vi "Spartan Server.vi"() -> ()   [LabVIEW 2011]
uses:
  server lib/Spartan Version.vi
  http/Spartan HTTP Server Globals.vi
  Addons/internet/http/http0.llb/HTTP LVHTTP Global.vi
  OpenG.LIB/file/file.llb/Convert File Extension (Path)__ogtk.vi
  server lib/Spartan CONFIG Global.vi
panel:
  out "Uptime":dbl
  in  "clear":bool
  in  "?":bool
  out "DD Queue":i32
  out "ver":string
  in  "Show Log":bool
  out "tall":bool
  out "wide":bool
  out "narrow":bool
  out "Log":string
  out "short":bool
  out "time up":string
  out "time":string
  in  "do stop":bool
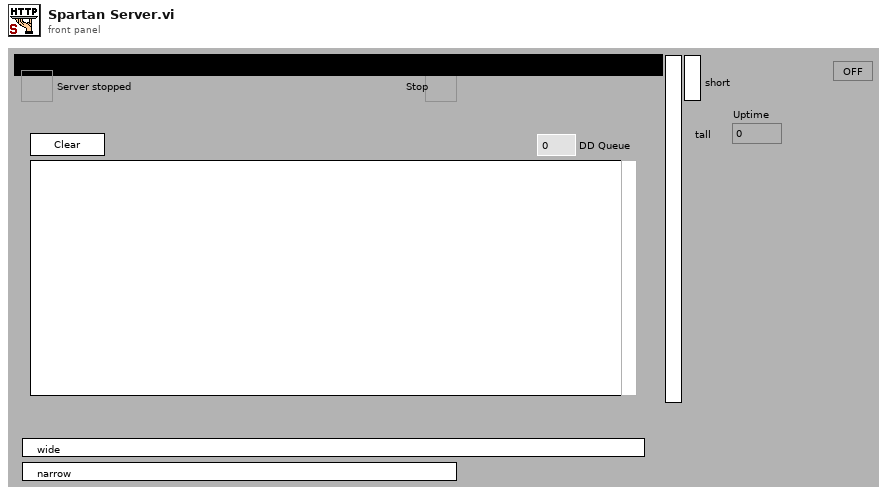
[diagram p1: front panel]
types:
  T1 = enum32{"Invalid", "Standard", "Closed", "Hidden", "Minimized", "Maximized"}
  T2 = enum32{"SW_SHOWDEFAULT", "SW_FORCEMINIMIZE", "SW_HIDE", "SW_MAXIMIZE", "SW_RESTORE", "SW_SHOW", "SW_SHOWMAXIMIZED", "SW_SHOWMINIMIZED", "SW_SHOWMINNOACTIVE", "SW_SHOWNA", "SW_SHOWNOACTIVATE", "SW_SHOWNORMAL"}
  T3 = typedef "OGAB Version.ctl" = cluster{"Version":string, "Build Number":u32, "Build Date/Time":dbl}
  T4 = typedef "DIAdem Queues.ctl" = cluster{"DIAdem Queue":refnum<queue>, "Datasheet Queue":refnum<queue>, "Runtest Queue":refnum<queue>}
  T5 = typedef "DIAdem Reference.ctl" = cluster{"ToCommand Reference":refnum<k7>, "ToDataSheet Reference":refnum<k7>}
  T6 = typedef "Semaphore RefNum" = refnum<k1>
  T7 = typedef "hWnd.ctl" = refnum<k1>
  T8 = typedef "siwutil32.ctl" = refnum<k7>
  T9 = typedef "LVRectTypeDef.ctl" = cluster{"left":i16, "top":i16, "right":i16, "bottom":i16}
  T10 = typedef "sizeaction.ctl" = enum32{"Minimized", "Maximized", "Resized"}
  T11 = typedef "Rendezvous RefNum" = refnum<k1>
  T12 = typedef "Keyed Array.ctl" = cluster{"keys":string[], "values":string[]}
  T13 = enum32{"invalid app kind", "Development System", "Run Time System", "Student Edition", "Embedded LabVIEW", "Evaluation", "Custom"}
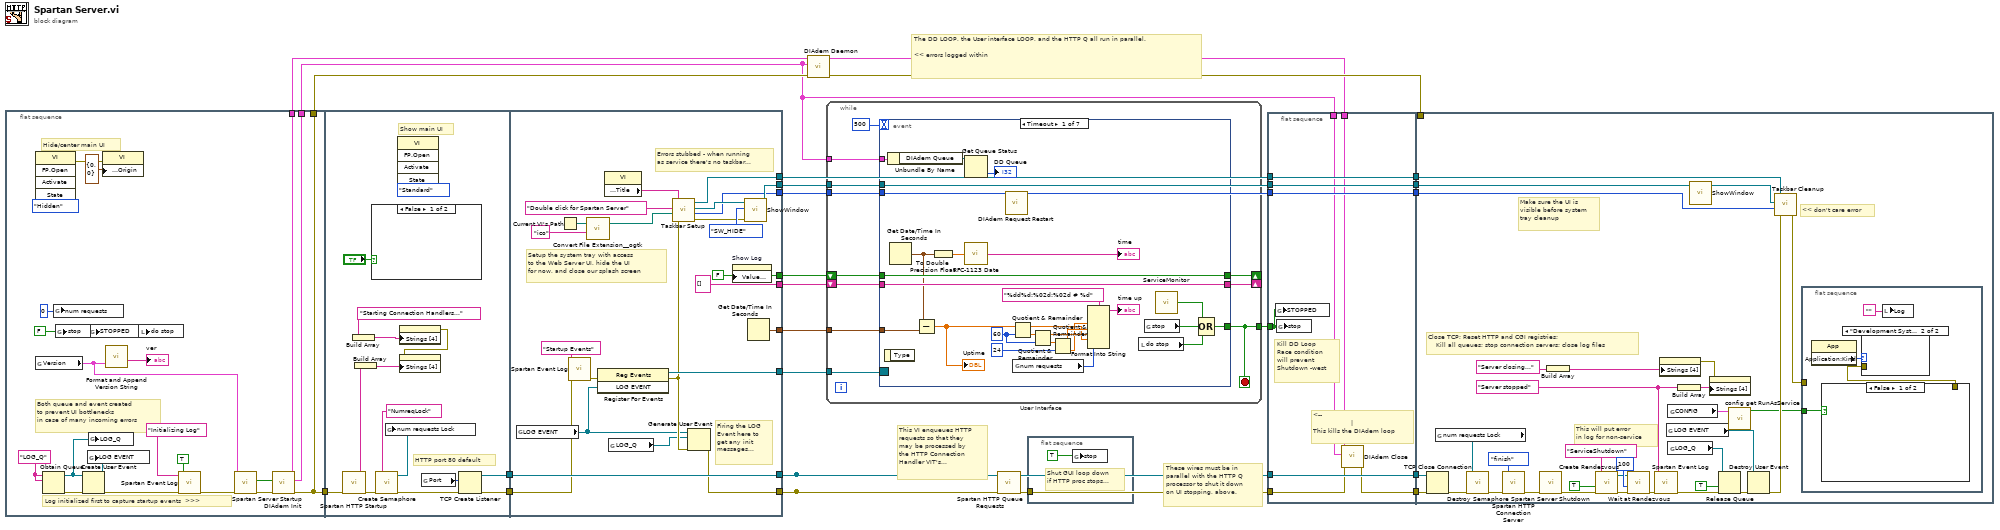
[diagram p0: block diagram]
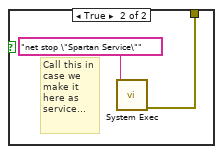
[diagram p2: hidden frame]
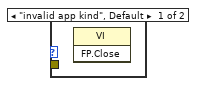
[diagram p3: hidden frame]
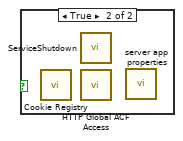
[diagram p4: hidden frame]
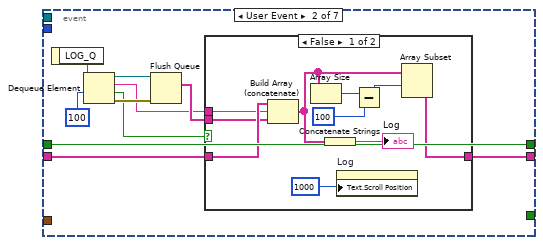
[diagram p5: hidden frame]
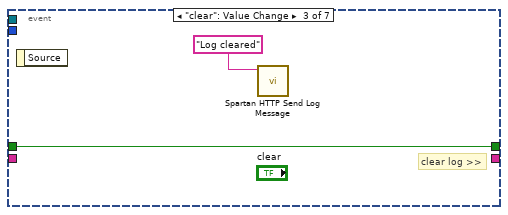
[diagram p7: hidden frame]
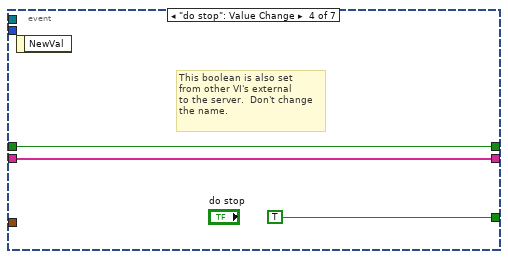
[diagram p8: hidden frame]
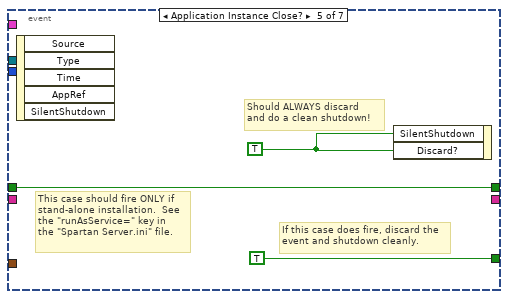
[diagram p9: hidden frame]
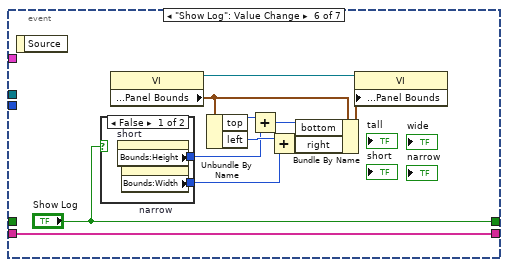
[diagram p10: hidden frame]
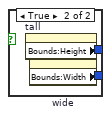
[diagram p11: hidden frame]
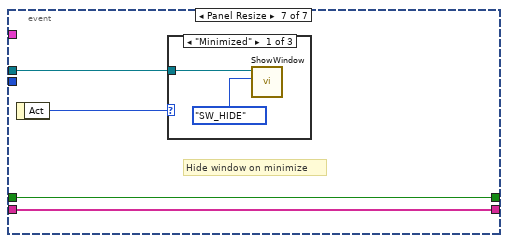
[diagram p12: hidden frame]
diagram:
  # "The DD LOOP, the User interface LOOP, and the HTTP Q all run in parallel.  \n\n<< errors logged within"
  # "These wires must be in\nparallel with the HTTP Q\nprocessor to shut it down\non UI stopping, above."
  # "This VI enqueues HTTP\nrequests so that they\nmay be processed by\nthe HTTP Connection\nHandler VIT's..."
  n1 = flat-sequence {
    tunnel: [w40] -> w12
    tunnel: [w42] -> w1
    tunnel: [w41] -> w3
    tunnel: [w40] -> w11
    tunnel: w12 -> [w50]
    tunnel: [w53] -> w18
    tunnel: [w51] -> w17
    tunnel: [w73] -> w22
    tunnel: [w81] -> w16
    tunnel: [w62] -> w13
    tunnel: [w80] -> w23
    tunnel: [w68] -> w10
    tunnel: w18 -> [w81]
    tunnel: [w76] -> w20
    tunnel: [w75] -> w21
    tunnel: [w74] -> w19
    tunnel: w17 -> [w61]
    tunnel: [string[] []] -> w14
    frame #0 {
      w32 = FALSE
      w36 = "LOG_Q"
      # "Hide/center main UI"
      # "Log initialized first to capture startup events  >>>"
      # "Both queue and event created\nto prevent UI bottlenecks\nin case of many incoming errors"
      n2 = invoke class="VI" method="FP.Open"("State"=T1."Hidden") -> (error out=w37:errorcluster)  [unwired: 4 in, 4 out]
      n3 = global read "Spartan Version.vi" "Version"() -> (w26:T3)
      n4 = Obtain Queue(name (unnamed)=w36, element data type=w36) -> (queue out=w33:refnum<queue>, error out=w35:errorcluster)  [unwired: 3 in, 1 out]
      n5 = global write "Spartan HTTP Server Globals.vi" "num requests"(u32 0 ("num requests")) -> ()
      n6 = global write "Spartan HTTP Server Globals.vi" "stop"(w32) -> ()
      n7 = Create User Event(user event datatype=w33, error in=w35) -> (user event=w34:refnum<user-event>, error out=w27:errorcluster)
      n8 = global write "Spartan HTTP Server Globals.vi" "LOG EVENT"(w34) -> ()
      n9 = global write "Spartan HTTP Server Globals.vi" "LOG_Q"(w33) -> ()
      n10 = global write "Spartan Version.vi" "STOPPED"(w32) -> ()
      n11 = property class="VI"(error in=w37, "Front Panel Window:Origin"=cluster{"Horizontal":i16, "Vertical":i16} {"Horizontal"=0, "Vertical"=0}) -> ()  [unwired: 1 in, 2 out]
      n12 = call "Format and Append Version String.vi"("Version"=w26) -> ("String with Version"=→"ver":string)  [unwired: 1 in, 9 out]
      n13 = local write "do stop"(w32) -> ()
      n14 = call "Spartan Event Log.vi"("Force Archive? (f)"=TRUE ("archive previous"), "error in (no error)"=w27, "message (\"\")"="Initializing Log" ("name (unnamed)")) -> ("error out"=w25:errorcluster)  [unwired: 2 in, 3 out]
      n15 = call "Spartan Server Startup.vi"("error in (no error)"=w25, "Version"=w26) -> ("error out"=w43:errorcluster, "DIAdem?"=w24:bool)  [unwired: 8 in]
      n16 = call "DIAdem Init.vi"("error in (no error)"=w43, "Startup DIAdem? (f)"=w24) -> ("error out"=w40:errorcluster, "Queues"=w41:T4, "DIAdem Reference"=w42:T5)  [unwired: 1 in, 6 out]
    }
    frame #1 {
      # "Show main UI"
      # "HTTP port 80 default"
      n17 = call "Spartan HTTP Startup.vi"("error in (no error)"=w50) -> ("error out"=w49:errorcluster, "Startup Message"=w55:string)  [unwired: 3 in, 2 out]
      n18 = Build Array("Starting Connection Handlers..." ("status")) -> (w56:string[])
      n19 = Build Array(w55) -> (w58:string[])
      n20 = case shown="False" "?" {
        frame False {
        }
        frame True {
          n21 = call "Cookie Registry.vi"() -> ()  [unwired: 4 in, 8 out]
          n22 = call "ServiceShutdown.vi"() -> ()  [unwired: 1 in, 1 out]
          n23 = call "HTTP Global ACF Access.vi"() -> ()  [unwired: 5 in, 7 out]
          n24 = call "server app properties.vi"() -> ()  [unwired: 9 in, 3 out]
        }
      }
      n25 = call <vilib>:"Create Semaphore.vi"("error in (no error)"=w49, "name (unnamed)"="NumreqLock" ("RegisterWindoMessage")) -> ("error out"=w46:errorcluster, "semaphore"=w47:T6)  [unwired: 1 in, 3 out]
      n26 = global write "Spartan HTTP Server Globals.vi" "num requests Lock"(w47) -> ()
      n27 = invoke class="VI" method="FP.Open"("State"=T1."Standard") -> ()  [unwired: 4 in, 5 out]
      n28 = property on="Show Log" class="Bool (strict)"("Strings [4]"=w56) -> (error out=w52:errorcluster)  [unwired: 2 in, 1 out]
      n29 = property on="Show Log" class="Bool (strict)"(error in=w52, "Strings [4]"=w58) -> ()  [unwired: 1 in, 2 out]
      n30 = global read "HTTP LVHTTP Global.vi" "Port"() -> (w54:u16)
      n31 = TCP Create Listener(8:w46, 10:w54) -> (0:w51:errorcluster, 3:w53:refnum<k5>)  [unwired: 4 out]
    }
    frame #2 {
      w80 = FALSE
      # "Firing the LOG\nEvent here to\nget any init\nmessages..."
      # "Setup the system tray with access\nto the Web Server UI, hide the UI\nfor now, and close our splash screen"
      # "Errors stubbed - when running\nas service there's no taskbar..."
      n32 = global read "Spartan HTTP Server Globals.vi" "LOG EVENT"() -> (w67:refnum<user-event>)
      n33 = Current VI's Path() -> (path=w65:path)
      n34 = call "Spartan Event Log.vi"("error in (no error)"=w61, "message (\"\")"="Startup Events" ("name (unnamed)")) -> ("error out"=w60:errorcluster)  [unwired: 3 in, 3 out]
      n35 = call-poly "Convert File Extension__ogtk.vi"("new ending (none)"="ico", "file name"=w65) -> ("new filename"=w63:path)  [unwired: 1 out]
      n36 = register-events(error in=w60, w67) -> (reference out=w73:refnum<event-registration>, error out=w69:errorcluster)  [unwired: 1 in]
      n37 = property class="VI"() -> ("Front Panel Window:Title"=w72:string)  [unwired: 2 in, 2 out]
      n38 = global read "Spartan HTTP Server Globals.vi" "LOG_Q"() -> (w66:refnum<queue>)
      n39 = call "Taskbar Setup.vi"("error in (no error)"=w69, "DEV Icon Path (empty)"=w63, "Tooltip Text (\"\")"="Double click for Spartan Server", "Window Name (\"\")"=w72) -> ("error out"=w78:errorcluster, "hIcon"=w74:i32, "hWnd"=w77:T7, "siwutil32"=w75:T8)
      n40 = Generate User Event(user event=w67, event data cluster=w66, error in=w69) -> (error out=w68:errorcluster)  [unwired: 1 out]
      n41 = property on="Show Log" class="Bool (strict)"("Value (Signaling)"=w80) -> ()  [unwired: 2 in, 2 out]
      n42 = call "ShowWindow.vi"("error in (no error)"=w78, "nCmdShow\n(SW_SHOWNORMAL)"=T2."SW_HIDE" ("nCmdShow\n(SW_SHOWNORMAL)"), "hWnd (NULL)"=w77) -> ("dup hWnd"=w76:T7)  [unwired: 8 out]
      n43 = Get Date/Time In Seconds() -> (seconds since 1Jan1904=w62:timestamp)
    }
  }
  n44 = call "DIAdem Daemon.vi"("error in (no error)"=w11, "Queues"=w3, "DIAdem Reference"=w1) -> ("error out"=w2:errorcluster)  [unwired: 8 out]
  n45 = while "User Interface" {
    shift-left: w23 -> [w92]
    shift-right: [w91] -> _
    tunnel: w13 -> [w90]
    tunnel: [w89] -> w4
    tunnel: w22 -> [w88]
    tunnel: w20 -> [w87]
    tunnel: w19 -> [w86]
    shift-right: [w85] -> _
    shift-left: w14 -> [w84]
    tunnel: w3 -> [w82]
    stop <- w89 stop-if-true
    n46 = event shown="[0] Timeout" {
      selector: w88 -> [_ _ _ _ _ _ _]
      dyn-events: _ -> [_ _ _ _ _ _ _]
      timeout: 500 -> [_ _ _ _ _ _ _]
      tunnel: w92 -> [w117 w127 w140 w143 w146 _ w164]
      tunnel: [w117 w127 w140 w143 w146 "Show Log" w164] -> w91
      tunnel: w90 -> [w104 _ _ _ _ _ _]
      tunnel: [w103 _ _ TRUE TRUE _ _] -> w89
      tunnel: w87 -> [_ _ _ _ _ _ w163]
      tunnel: w86 -> [_ _ _ _ _ _ _]
      tunnel: [w100 w119 _ w142 _ w147 w162] -> w85
      tunnel: w84 -> [w100 w118 _ w142 _ w147 w162]
      tunnel: w82 -> [w98 _ _ _ _ _ _]
      event Timeout {
        w111 = 60 ("y")
        n47 = event-data() -> ()  [unwired: 2 out]
        n48 = Unbundle By Name(w98) -> ("DIAdem Queue"=w93:refnum<queue>)
        n49 = Get Date/Time In Seconds() -> (seconds since 1Jan1904=w96:timestamp)
        n50 = Subtract(x=w96, y=w104) -> (x-y=w109:dbl)
        "Uptime" <- w109
        n51 = To Double Precision Float(number=w96) -> (double precision float=w95:dbl)
        n52 = Get Queue Status(queue=w93) -> (# elements in queue=→"DD Queue":i32)  [unwired: 1 in, 8 out]
        n53 = call "RFC-1123 Date.vi"("time (now)"=w95) -> ("GMT Date/Time"=→"time":string)  [unwired: 1 in]
        n54 = call "DIAdem Request Restart.vi"() -> ()  [unwired: 3 in, 9 out]
        n55 = Quotient & Remainder(x=w109, y=w111) -> (x-y*floor(x/y)=w106:dbl, floor(x/y)=w115:dbl)
        n56 = global read "Spartan HTTP Server Globals.vi" "num requests"() -> (w105:u32)
        n57 = Quotient & Remainder(x=w115, y=w111) -> (x-y*floor(x/y)=w114:dbl, floor(x/y)=w110:dbl)
        n58 = Quotient & Remainder(x=w110, y=24) -> (x-y*floor(x/y)=w113:dbl, floor(x/y)=w112:dbl)
        n59 = Format Into String(format string="%dd%d:%02d:%02d # %d", w112, w113, w114, w106, w105) -> (resulting string=→"time up":string)  [unwired: 2 in, 1 out]
        n60 = local read "do stop"() -> (w101:bool)
        n61 = global read "Spartan HTTP Server Globals.vi" "stop"() -> (w102:bool)
        n62 = call "ServiceMonitor.vi"() -> ("Stop?"=w97:bool)  [unwired: 1 in]
        n63 = Compound Arithmetic op=OR(w97, w102, w101) -> (w103:bool)
      }
      event User Event {
        n64 = event-data() -> ("LOG_Q"=w124:refnum<queue>)  [unwired: 1 out]
        n65 = Dequeue Element(queue=w124, timeout in ms (-1)=100) -> (queue out=w125:refnum<queue>, element=w121:string, timed out?=w120:bool, error out=w126:errorcluster)  [unwired: 1 in]
        n66 = Flush Queue(queue=w125, error in (no error)=w126) -> (remaining elements=w122:string[])  [unwired: 2 out]
        n67 = case shown="False" w120 {
          tunnel: w118 -> [w135 w138]
          tunnel: w122 -> [w134 _]
          tunnel: w121 -> [w133 _]
          tunnel: [w137 w138] -> w119
          frame False {
            n68 = Build Array (concatenate)(w135, w133, w134) -> (w129:string[])
            n69 = Array Size(array=w129) -> (size(s)=w132:i32)
            n70 = Concatenate Strings(w129) -> (→"Log":string)
            n71 = property on="Log" class="Str"("Text.Scroll Position"=u32 1000 ("Scroll Position")) -> ()  [unwired: 2 in, 2 out]
            n72 = Subtract(x=w132, y=100) -> (x-y=w136:i32)
            n73 = Array Subset(array=w129, index=w136) -> (w137:string[])  [unwired: 1 in]
          }
          frame True {
          }
        }
      }
      event "clear": Value Change {
        # "clear log >>"
        n74 = event-data() -> ()  [unwired: 2 out]
        n75 = call "Spartan HTTP Send Log Message.vi"("message"="Log cleared") -> ()  [unwired: 7 out]
      }
      event "do stop": Value Change {
        # "This boolean is also set\nfrom other VI's external\nto the server.  Don't change\nthe name."
        n76 = event-data() -> ()  [unwired: 2 out]
      }
      event Application Instance Close? {
        w145 = TRUE
        # "If this case does fire, discard the\nevent and shutdown cleanly."
        # "This case should fire ONLY if\nstand-alone installation.  See\nthe \"runAsService=\" key in\nthe \"Spartan Server.ini\" file."
        # "Should ALWAYS discard\nand do a clean shutdown!"
        n77 = event-data() -> ()  [unwired: 6 out]
        n78 = event-data("SilentShutdown"=w145, "Discard?"=w145) -> ()  [unwired: 1 in, 1 out]
      }
      event "Show Log": Value Change {
        n79 = event-data() -> ()  [unwired: 2 out]
        n80 = case shown="False" "Show Log" {
          tunnel: [w159 w161] -> w151
          tunnel: [w158 w160] -> w155
          frame False {
            n81 = property on="short" class="Bool (strict)"() -> ("Bounds:Height"=w159:u32)  [unwired: 2 in, 2 out]
            n82 = property on="narrow" class="Bool (strict)"() -> ("Bounds:Width"=w158:u32)  [unwired: 2 in, 2 out]
          }
          frame True {
            n83 = property on="tall" class="Bool (strict)"() -> ("Bounds:Height"=w161:u32)  [unwired: 2 in, 2 out]
            n84 = property on="wide" class="Bool (strict)"() -> ("Bounds:Width"=w160:u32)  [unwired: 2 in, 2 out]
          }
        }
        n85 = property class="VI"() -> (reference out=w157:refnum<vi>, "Front Panel Window:Panel Bounds"=w156:T9)  [unwired: 2 in, 1 out]
        n86 = Unbundle By Name(w156) -> ("top"=w152:i16, "left"=w153:i16)
        n87 = Add(x=w152, y=w151) -> (x+y=w149:u32)
        n88 = Add(x=w153, y=w155) -> (x+y=w154:u32)
        n89 = Bundle By Name(cluster=w156, "bottom"=w149, "right"=w154) -> (w150:T9)
        n90 = property class="VI"(reference=w157, "Front Panel Window:Panel Bounds"=w150) -> ()  [unwired: 1 in, 2 out]
      }
      event Panel Resize {
        # "Hide window on minimize"
        n91 = event-data() -> ("Act"=w165:T10)  [unwired: 1 out]
        n92 = case shown="\"Minimized\"" w165 {
          tunnel: w163 -> [w166 _ _]
          frame "Minimized" {
            n93 = call "ShowWindow.vi"("nCmdShow\n(SW_SHOWNORMAL)"=T2."SW_HIDE" ("nCmdShow\n(SW_SHOWNORMAL)"), "hWnd (NULL)"=w166) -> ()  [unwired: 1 in, 9 out]
          }
          frame "Maximized" {
          }
          frame "Resized" {
          }
        }
      }
    }
  }
  n94 = call "Spartan HTTP Queue Requests.vi"("error in (no error)"=w10, "Listener ID"=w16) -> ("error out"=w15:errorcluster)  [unwired: 5 out]
  n95 = flat-sequence {
    tunnel: w15 -> [_]
    frame #0 {
      # "Shut GUI loop down\nif HTTP proc stops..."
      n96 = global write "Spartan HTTP Server Globals.vi" "stop"(TRUE) -> ()
    }
  }
  n97 = flat-sequence {
    tunnel: w4 -> [w173]
    tunnel: w10 -> [w170]
    tunnel: w19 -> [w174]
    tunnel: w20 -> [w175]
    tunnel: w21 -> [w176]
    tunnel: w16 -> [w177]
    tunnel: [w177] -> w9
    tunnel: [w176] -> w8
    tunnel: [w175] -> w7
    tunnel: [w174] -> w6
    tunnel: [w169] -> w5
    tunnel: w3 -> [w172]
    tunnel: w1 -> [w171]
    tunnel: w9 -> [w209]
    tunnel: w8 -> [w196]
    tunnel: w7 -> [w195]
    tunnel: w6 -> [w194]
    tunnel: w5 -> [w208]
    tunnel: w2 -> [_]
    frame #0 {
      # "<--\n                   |\nThis kills the DIAdem loop"
      # "Kill DD Loop\nRace condition\nwill prevent\nShutdown -west"
      n98 = global write "Spartan Version.vi" "STOPPED"(w173) -> ()
      n99 = global write "Spartan HTTP Server Globals.vi" "stop"(w173) -> ()
      n100 = call "DIAdem Close.vi"("error in (no error)"=w170, "DD queue"=w172, "DIAdem Reference"=w171) -> ("error out"=w169:errorcluster)  [unwired: 8 out]
    }
    frame #1 {
      w190 = "Server stopped" ("name (unnamed)")
      # "This will put error\nin log for non-service"
      # "<< don't care error"
      # "Make sure the UI is\nvisible before system\ntray cleanup"
      # "Close TCP; Reset HTTP and CGI registries;  \n    Kill all queues; stop connection servers; close log files"
      n101 = TCP Close Connection(connection ID=w209, error in (no error)=w208) -> (error out=w200:errorcluster)  [unwired: 2 out]
      n102 = global read "Spartan HTTP Server Globals.vi" "num requests Lock"() -> (w193:T6)
      n103 = call <vilib>:"Destroy Semaphore.vi"("error in (no error)"=w200, "semaphore"=w193) -> ("error out"=w203:errorcluster)  [unwired: 5 out]
      n104 = call "Spartan HTTP Connection Server.vi"("error in (no error)"=w203, "function (init)"=enum16{"init", "finish"}."finish") -> ("error out"=w198:errorcluster)  [unwired: 1 in, 4 out]
      n105 = call "Spartan Server Shutdown.vi"("error in (no error)"=w198) -> ("error out"=w179:errorcluster)  [unwired: 1 in, 5 out]
      n106 = Build Array("Server closing..." ("status")) -> (w205:string[])
      n107 = call <vilib>:"Create Rendezvous.vi"("error in (no error)"=w179, "return existing (F)"=TRUE, "name (unnamed)"="ServiceShutdown") -> ("error out"=w184:errorcluster, "rendezvous"=w181:T11)  [unwired: 2 in, 1 out]
      n108 = call <vilib>:"Wait at Rendezvous.vi"("error in (no error)"=w184, "ms timeout (-1)"=100, "rendezvous"=w181) -> ("error out"=w178:errorcluster)  [unwired: 2 in, 2 out]
      n109 = call "Spartan Event Log.vi"("error in (no error)"=w178, "message (\"\")"=w190) -> ("error out"=w188:errorcluster)  [unwired: 3 in, 3 out]
      n110 = property on="Show Log" class="Bool (strict)"("Strings [4]"=w205) -> (error out=w189:errorcluster)  [unwired: 2 in, 1 out]
      n111 = global read "Spartan HTTP Server Globals.vi" "LOG EVENT"() -> (w201:refnum<user-event>)
      n112 = global read "Spartan CONFIG Global.vi" "CONFIG"() -> (w186:T12)
      n113 = global read "Spartan HTTP Server Globals.vi" "LOG_Q"() -> (w206:refnum<queue>)
      n114 = Build Array(w190) -> (w191:string[])
      n115 = call "ShowWindow.vi"("hWnd (NULL)"=w195) -> ("dup hWnd"=w197:T7)  [unwired: 2 in, 8 out]
      n116 = property on="Show Log" class="Bool (strict)"(error in=w189, "Strings [4]"=w191) -> ()  [unwired: 1 in, 2 out]
      n117 = Release Queue(queue=w206, force destroy? (F)=TRUE, error in (no error)=w188) -> (error out=w199:errorcluster)  [unwired: 2 out]
      n118 = call "config get RunAsService.vi"("Config Keys"=w186) -> ("RunAsService?"=w185:bool)  [unwired: 4 out]
      n119 = Destroy User Event(user event=w201, error in=w199) -> (error out=w187:errorcluster)
      n120 = call "Taskbar Cleanup.vi"("error in (no error)"=w187, "hIcon"=w194, "hWnd"=w197, "siwutil32"=w196) -> ("error out"=w192:errorcluster)  [unwired: 3 out]
      n121 = flat-sequence {
        tunnel: w192 -> [_]
        tunnel: w185 -> [w210]
        frame #0 {
          n122 = property class="App"() -> ("Application:Kind"=w212:T13)  [unwired: 2 in, 2 out]
          n123 = case shown="False" w210 {
            tunnel: [_ w214] -> w211
            frame False {
            }
            frame True {
              # "Call this in\ncase we\nmake it \nhere as\nservice..."
              n124 = call <vilib>:"System Exec.vi"("command line"="net stop \"Spartan Service\"") -> ("error out"=w214:errorcluster)  [unwired: 7 in, 3 out]
            }
          }
          n125 = case shown="\"Development System\"" w212 {
            tunnel: w211 -> [_ _]
            frame "invalid app kind", Default {
              n126 = invoke class="VI" method="FP.Close"() -> ()  [unwired: 3 in, 3 out]
            }
            frame "Development System" {
            }
          }
          n127 = local write "Log"("") -> ()
        }
      }
    }
  }
